vi "GetRPMSubVI.vi"(9 "Range":dbl(slide) scale=9.0..14.0, 10 "array type (2D Dbl)":dbl[](array[numeric]), 11 "array type (2D Dbl) 2":dbl[][](array[numeric])) -> (2 "Array Index":dbl, 3 "RPM Output":dbl)   [LabVIEW 2019]
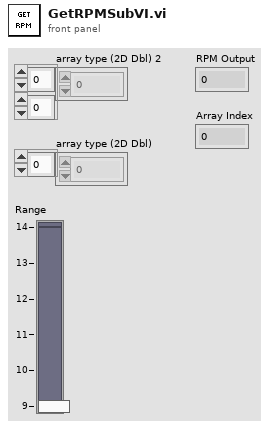
[diagram p1: front panel]
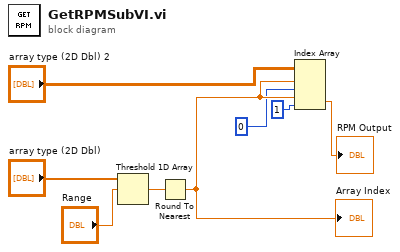
[diagram p0: block diagram]
diagram:
  n1 = Threshold 1D Array(2:"Range", 3:"array type (2D Dbl)") -> (0:w3:dbl)  [unwired: 1 in]
  n2 = Round To Nearest(number=w3) -> (nearest integer value=w7:dbl)
  "Array Index" <- w7
  n3 = Index Array(array="array type (2D Dbl) 2", index (row) #1=w7, index (col) #1=0 ("disabled index (col)"), index (row) #2=w7, index (col) #2=1 ("index (col)")) -> (element #2=→"RPM Output":dbl)  [unwired: 1 out]
